vi "Periodic Tasks.vi"(8 "error in":errorcluster) -> ()   [LabVIEW 2014]
doc: "This VI runs in parallel to other tasks. It can contain as many user-defined periodic loops as you need. These can carry out PID or other sorts of timed response."
uses:
  <vilib>/Rock Robotics/WPI/Relay/WPI_RelayValue.ctl
  <vilib>/Rock Robotics/SystemInterfaces/Utilities/FPGA_UtilitiesLED Source.ctl
  <vilib>/Rock Robotics/SystemInterfaces/Utilities/FPGA_UtilitiesLED State.ctl
  <vilib>/Rock Robotics/WPI/DriverStation/WPI_DriverStationRobotMode2.ctl
  <vilib>/Rock Robotics/WPI/Compressor/WPI_CompressorGetSetRefNum.vi
  Robot Global Data.vi
  <vilib>/Rock Robotics/WPI/Solenoid/Deprecated/WPI_SolenoidSetBool.vi
panel:
  out "Passing Ball":bool
  out "kicker was on":bool
  out "Lights Relay Indicator":T1
  out "pickup arm motor shooting":bool
  out "Gate shooting":bool
  out "Catapult Switch Triggered":bool
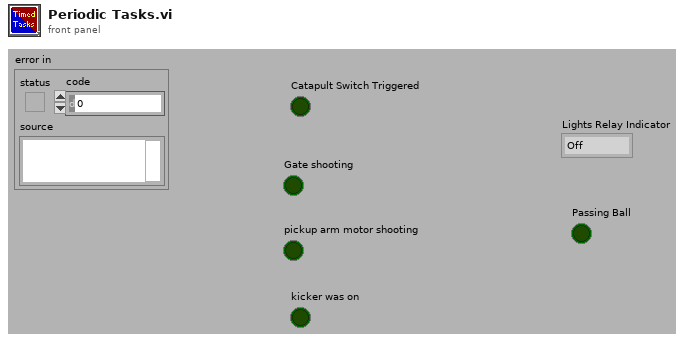
[diagram p1: front panel]
types:
  T1 = typedef "WPI_RelayValue.ctl" = enum16{"Off", "On", "Forward", "Reverse"}
  T2 = typedef "WPI_RelayDevRef.ctl" = cluster{"DevStatus":errorcluster, "Relay Channel":T3, "Digital Module":T4, "Relay Direction":T5}
  T3 = typedef "FPGA_DIORelayChannel.ctl" = enum8{"Relay 1", "Relay 2", "Relay 3", "Relay 4", "Relay 5", "Relay 6", "Relay 7", "Relay 8", "Invalid"}
  T4 = typedef "FPGA_TypedefDigitalModule.ctl" = enum16{"Digital Module 1", "Digital Module 2"}
  T5 = typedef "WPI_RelayDirection.ctl" = enum16{"Both directions", "Forward only", "Reverse only"}
  T6 = typedef "WPI_DigitalInputDevRef.ctl" = cluster{"DevStatus":errorcluster, "DIO Channel":T7, "Digital Module":T4}
  T7 = typedef "FPGA_DIOChannel.ctl" = enum8{"DIO 1", "DIO 2", "DIO 3", "DIO 4", "DIO 5", "DIO 6", "DIO 7", "DIO 8", "DIO 9", "DIO 10", "DIO 11", "DIO 12", "DIO 13", "DIO 14", "Invalid"}
  T8 = typedef "WPI_SolenoidDevRef.ctl" = cluster{"DevStatus":errorcluster, "Solenoid Module":T9, "Forward Solenoid Channel":T10, "Reverse Solenoid Channel":T10}
  T9 = typedef "FPGA_TypedefSolenoidModule.ctl" = enum16{"Solenoid Module 1", "Solenoid Module 2"}
  T10 = typedef "WPI_SolenoidChannel.ctl" = enum8{"Solenoid 1", "Solenoid 2", "Solenoid 3", "Solenoid 4", "Solenoid 5", "Solenoid 6", "Solenoid 7", "Solenoid 8", "Invalid"}
  T11 = typedef "WPI_MotorControlDeviceRef.ctl" = cluster{"DeviceStatus":errorcluster, "Type":enum16{"PWM", "CAN"}, "PWM":cluster{"Digital Module":T4, "PWM Channel":T12, "DeadBand":T13}, "CAN":cluster{"Device Number":u8, "Control Mode":T14, "Semaphore":T15, "Max Vout":dbl}, "Invert":bool, "TransformRef":T16, "InvTransformRef":T16}
  T12 = typedef "FPGA_DIOPWMChannel.ctl" = enum8{"PWM 1", "PWM 2", "PWM 3", "PWM 4", "PWM 5", "PWM 6", "PWM 7", "PWM 8", "PWM 9", "PWM 10", "Invalid"}
  T13 = typedef "WPI_PWMDeadband.ctl" = cluster{"Name":string, "maxPositivePwm":i32, "minPositivePwm":i32, "centerPwm":i32, "maxNegativePwm":i32, "minNegativePwm":i32, "angularRange":u16}
  T14 = typedef "WPI_CANJaguar_ControlMode.ctl" = enum8{"Percent VBus", "Current", "Speed", "Position", "Voltage"}
  T15 = typedef "Semaphore RefNum" = refnum<k1>
  T16 = typedef "WPI_PWMTransform_ConPane.ctl" = refnum<vi>
  T17 = typedef "WPI_AnalogChannelDevRef.ctl" = cluster{"DevStatus":errorcluster, "Analog Module":T18, "Analog Channel":T19}
  T18 = typedef "FPGA_TypedefAnalogModule.ctl" = enum16{"Analog Module 1", "Analog Module 2"}
  T19 = typedef "FPGA_AIChannel.ctl" = enum8{"AI 1", "AI 2", "AI 3", "AI 4", "AI 5", "AI 6", "AI 7", "AI 8", "Invalid"}
  T20 = typedef "FPGA_UtilitiesLED State.ctl" = enum16{"Off", "On", "Toggle"}
  T21 = typedef "FPGA_UtilitiesLED Source.ctl" = enum16{"User LED", "FPGA LED"}
  T22 = typedef "WPI_DriverStationRobotMode2.ctl" = enum16{"Autonomous Disabled", "Autonomous Enabled", "Teleop Disabled", "Teleop Enabled", "Disconnected", "Finish", "Test Disabled", "Test Enabled"}
  T23 = typedef "WPI_CompressorDevRef.ctl" = cluster{"DevStatus":errorcluster, "DigitalInputDevRef":T6, "RelayDevRef":T2}
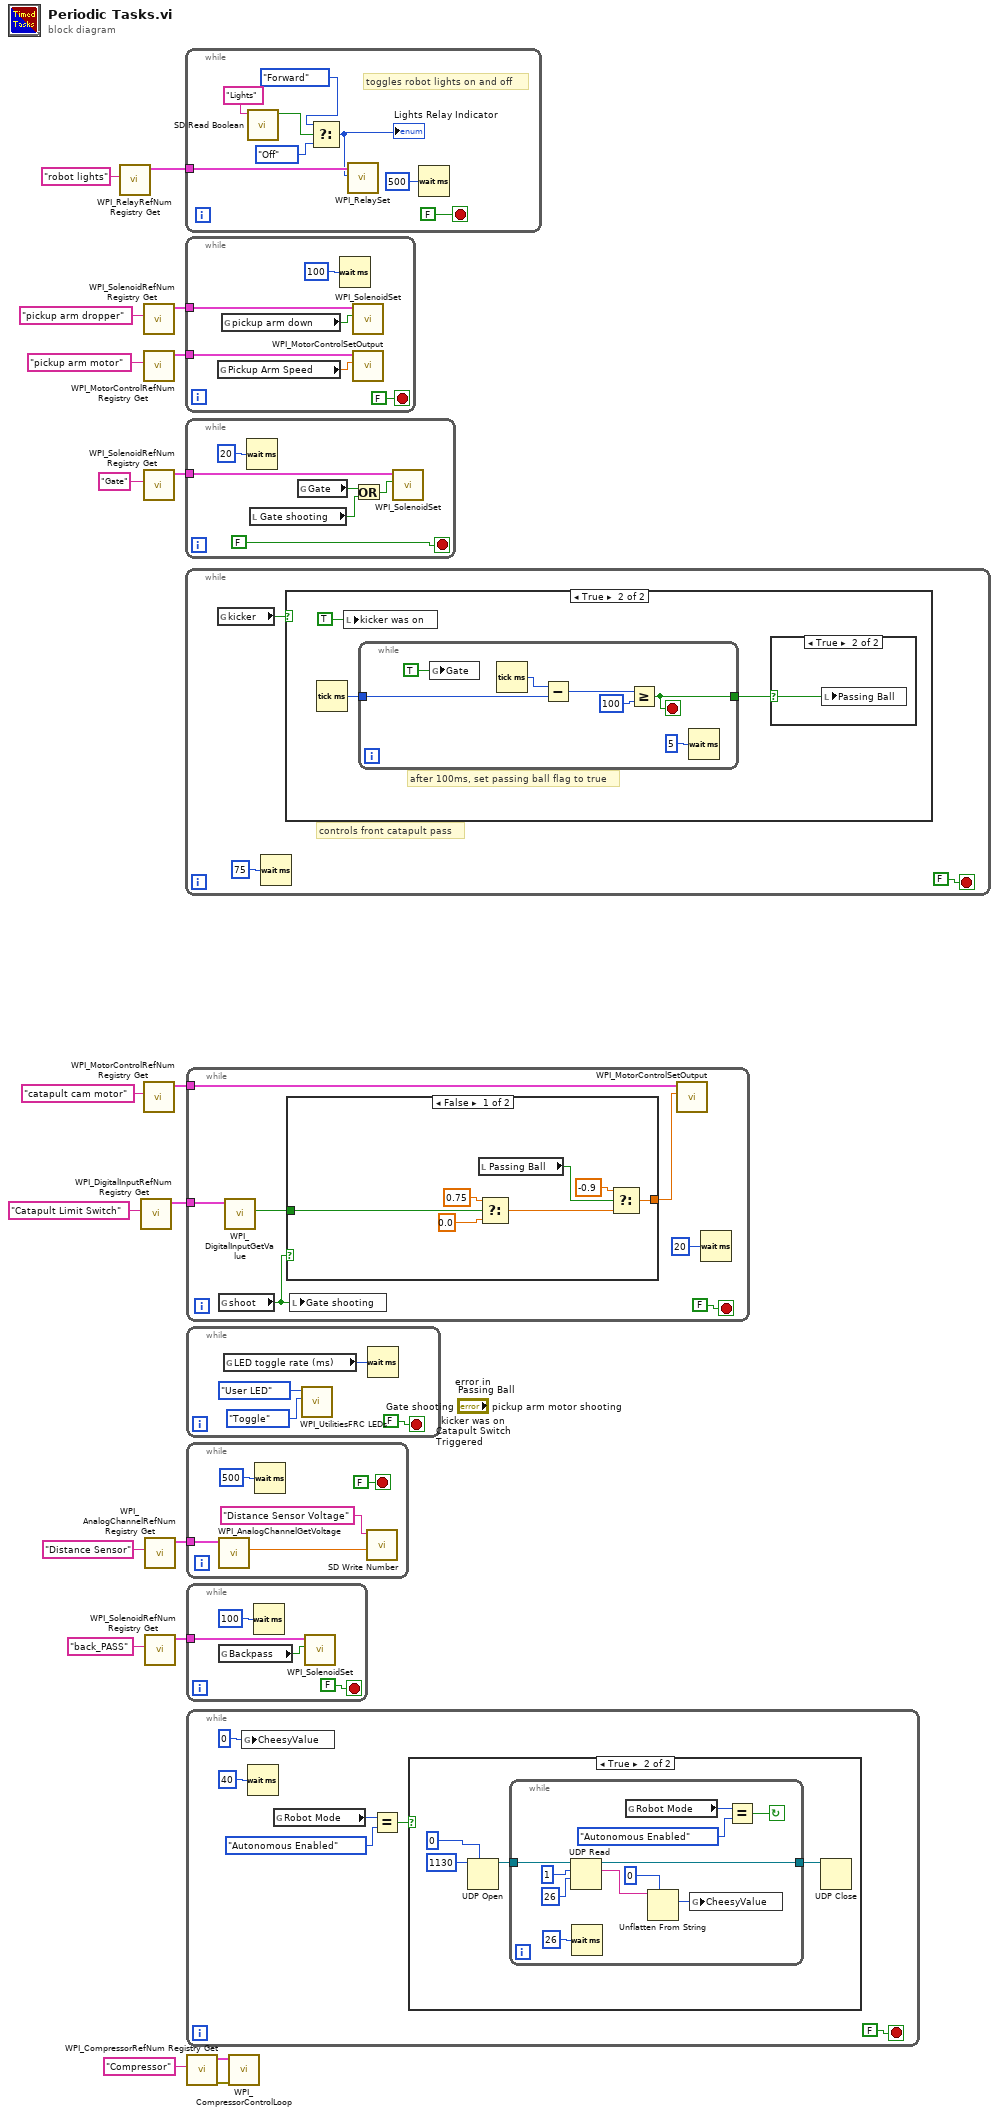
[diagram p0: block diagram]
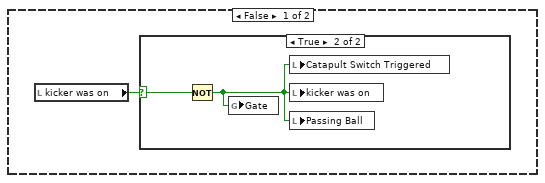
[diagram p3: hidden frame]
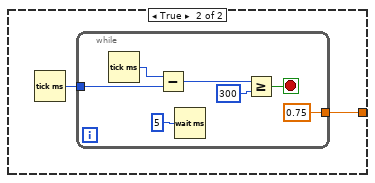
[diagram p6: hidden frame]
diagram:
  n1 = call <vilib>:"WPI_RelayRefNum Registry Get.vi"("refnum name"="robot lights") -> ("RelayDevRef"=w6:T2)  [unwired: 9 in, 1 out]
  n2 = call <vilib>:"WPI_DigitalInputRefNum Registry Get.vi"("refnum name"="Catapult Limit Switch") -> ("DigitalInputDevRef"=w8:T6)  [unwired: 9 in, 1 out]
  n3 = call <vilib>:"WPI_SolenoidRefNum Registry Get.vi"("refnum name"="pickup arm dropper") -> ("SolenoidDevRef"=w12:T8)  [unwired: 9 in, 1 out]
  n4 = call <vilib>:"WPI_MotorControlRefNum Registry Get.vi"("refnum name"="pickup arm motor") -> ("MotorControlDevRef"=w10:T11)  [unwired: 9 in, 1 out]
  n5 = call <vilib>:"WPI_SolenoidRefNum Registry Get.vi"("refnum name"="Gate") -> ("SolenoidDevRef"=w5:T8)  [unwired: 9 in, 1 out]
  n6 = call <vilib>:"WPI_MotorControlRefNum Registry Get.vi"("refnum name"="catapult cam motor") -> ("MotorControlDevRef"=w15:T11)  [unwired: 9 in, 1 out]
  n7 = call <vilib>:"WPI_AnalogChannelRefNum Registry Get.vi"("refnum name"="Distance Sensor") -> ("AIDeviceRef"=w1:T17)  [unwired: 9 in, 1 out]
  n8 = call <vilib>:"WPI_SolenoidRefNum Registry Get.vi"("refnum name"="back_PASS") -> ("SolenoidDevRef"=w3:T8)  [unwired: 9 in, 1 out]
  n9 = while {
    tunnel: w6 -> [w24]
    stop <- FALSE stop-if-true
    # "toggles robot lights on and off"
    n10 = call <vilib>:"SD Read Boolean.vi"("Name"="Lights") -> ("Boolean"=w23:bool)  [unwired: 8 in, 2 out]
    n11 = Select(t=WPI_RelayValue."Forward" ("RelayValue"), s=w23, f=WPI_RelayValue."Off" ("RelayValue")) -> (s? t:f=w20:T1)
    "Lights Relay Indicator" <- w20
    n12 = call <vilib>:"WPI_RelaySet.vi"("RelayValue"=w20, "RelayDevRef"=w24) -> ()  [unwired: 8 in, 2 out]
    n13 = Wait (ms)(milliseconds to wait=u32 500) -> ()  [unwired: 1 out]
  }
  n14 = while {
    tunnel: w12 -> [w33]
    tunnel: w10 -> [w32]
    stop <- FALSE stop-if-true
    n15 = global read "Robot Global Data.vi" "Pickup Arm Speed"() -> (w29:dbl)
    n16 = global read "Robot Global Data.vi" "pickup arm down"() -> (w28:bool)
    n17 = Wait (ms)(milliseconds to wait=u32 100) -> ()  [unwired: 1 out]
    n18 = call-poly <vilib>:"WPI_SolenoidSet.vi"("Value"=w28, "SolenoidDevRef"=w33) -> ()  [unwired: 8 in, 2 out]
    n19 = call <vilib>:"WPI_MotorControlSetOutput.vi"("Output"=w29, "MotorControlDevRef"=w32) -> ()  [unwired: 7 in, 3 out]
  }
  n20 = while {
    tunnel: w5 -> [w35]
    stop <- FALSE stop-if-true
    n21 = Wait (ms)(milliseconds to wait=u32 20) -> ()  [unwired: 1 out]
    n22 = local read "Gate shooting"() -> (w39:bool)
    n23 = global read "Robot Global Data.vi" "Gate"() -> (w38:bool)
    n24 = Or(x=w38, y=w39) -> (x .or. y?=w34:bool)
    n25 = call-poly <vilib>:"WPI_SolenoidSet.vi"("Value"=w34, "SolenoidDevRef"=w35) -> ()  [unwired: 8 in, 2 out]
  }
  n26 = while {
    stop <- FALSE stop-if-true
    # "controls front catapult pass"
    n27 = global read "Robot Global Data.vi" "kicker"() -> (w40:bool)
    n28 = Wait (ms)(milliseconds to wait=u32 75) -> ()  [unwired: 1 out]
    n29 = case shown="True" w40 {
      frame False {
        n30 = local read "kicker was on"() -> (w43:bool)
        n31 = case shown="True" w43 {
          selector: w43 -> [_ w45]
          frame False {
          }
          frame True {
            n32 = Not(x=w45) -> (.not. x?=w44:bool)
            n33 = global write "Robot Global Data.vi" "Gate"(w44) -> ()
            n34 = local write "Catapult Switch Triggered"(w44) -> ()
            n35 = local write "kicker was on"(w44) -> ()
            n36 = local write "Passing Ball"(w44) -> ()
          }
        }
      }
      frame True {
        # "after 100ms, set passing ball flag to true"
        n37 = Tick Count (ms)() -> (millisecond timer value=w47:u32)
        n38 = local write "kicker was on"(TRUE ("kicker was on")) -> ()
        n39 = while {
          tunnel: w47 -> [w55]
          tunnel: [w50] -> w46
          stop <- w50 stop-if-true
          n40 = global write "Robot Global Data.vi" "Gate"(TRUE ("Gate")) -> ()
          n41 = Tick Count (ms)() -> (millisecond timer value=w54:u32)
          n42 = Subtract(x=w54, y=w55) -> (x-y=w53:u32)
          n43 = Greater Or Equal?(x=w53, y=u32 100) -> (x >= y?=w50:bool)
          n44 = Wait (ms)(milliseconds to wait=u32 5) -> ()  [unwired: 1 out]
        }
        n45 = case shown="True" w46 {
          selector: w46 -> [_ w56]
          frame False {
          }
          frame True {
            n46 = local write "Passing Ball"(w56) -> ()
          }
        }
      }
    }
  }
  n47 = while {
    tunnel: w15 -> [w61]
    tunnel: w8 -> [w59]
    stop <- FALSE stop-if-true
    n48 = global read "Robot Global Data.vi" "shoot"() -> (w57:bool)
    n49 = call <vilib>:"WPI_DigitalInputGetValue.vi"("DigitalInputDevRef"=w59) -> ("Value"=w58:bool)  [unwired: 8 in, 2 out]
    n50 = case shown="False" w57 {
      tunnel: [w70 w71] -> w60
      tunnel: w58 -> [w64 _]
      frame False {
        n51 = local read "Passing Ball"() -> (w69:bool)
        n52 = Select(t=0.75 ("f"), s=w64, f=0.0 ("t")) -> (s? t:f=w67:dbl)
        n53 = Select(t=-0.9, s=w69, f=w67) -> (s? t:f=w70:dbl)
      }
      frame True {
        n54 = Tick Count (ms)() -> (millisecond timer value=w72:u32)
        n55 = while {
          tunnel: [0.75 ("Output")] -> w71
          tunnel: w72 -> [w77]
          stop <- w74 stop-if-true
          n56 = Tick Count (ms)() -> (millisecond timer value=w78:u32)
          n57 = Subtract(x=w78, y=w77) -> (x-y=w73:u32)
          n58 = Wait (ms)(milliseconds to wait=u32 5) -> ()  [unwired: 1 out]
          n59 = Greater Or Equal?(x=w73, y=u32 300) -> (x >= y?=w74:bool)
        }
      }
    }
    n60 = local write "Gate shooting"(w57) -> ()
    n61 = call <vilib>:"WPI_MotorControlSetOutput.vi"("Output"=w60, "MotorControlDevRef"=w61) -> ()  [unwired: 7 in, 3 out]
    n62 = Wait (ms)(milliseconds to wait=u32 20) -> ()  [unwired: 1 out]
  }
  n63 = while {
    stop <- FALSE stop-if-true
    n64 = global read "Robot Global Data.vi" "LED toggle rate (ms)"() -> (w80:u32)
    n65 = call <vilib>:"WPI_UtilitiesFRC LEDs.vi"("State"=FPGA_UtilitiesLED_State."Toggle", "LED Type"=FPGA_UtilitiesLED_Source."User LED") -> ()  [unwired: 1 in, 9 out]
    n66 = Wait (ms)(milliseconds to wait=w80) -> ()  [unwired: 1 out]
  }
  n67 = while {
    tunnel: w1 -> [w86]
    stop <- FALSE stop-if-true
    n68 = call <vilib>:"WPI_AnalogChannelGetVoltage.vi"("AIDeviceRef"=w86) -> ("Voltage"=w85:dbl)  [unwired: 8 in, 2 out]
    n69 = Wait (ms)(milliseconds to wait=u32 500) -> ()  [unwired: 1 out]
    n70 = call <vilib>:"SD Write Number.vi"("Numeric"=w85, "Name"="Distance Sensor Voltage") -> ()  [unwired: 8 in, 2 out]
  }
  n71 = while {
    tunnel: w3 -> [w90]
    stop <- FALSE stop-if-true
    n72 = global read "Robot Global Data.vi" "Backpass"() -> (w89:bool)
    n73 = Wait (ms)(milliseconds to wait=u32 100) -> ()  [unwired: 1 out]
    n74 = call-poly <vilib>:"WPI_SolenoidSet.vi"("Value"=w89, "SolenoidDevRef"=w90) -> ()  [unwired: 8 in, 2 out]
  }
  n75 = while {
    stop <- FALSE stop-if-true
    n76 = global write "Robot Global Data.vi" "CheesyValue"(u8 0 ("CheesyValue")) -> ()
    n77 = Wait (ms)(milliseconds to wait=u32 40) -> ()  [unwired: 1 out]
    n78 = global read "Robot Global Data.vi" "Robot Mode"() -> (w94:T22)
    n79 = Equal?(x=w94, y=WPI_DriverStationRobotMode2."Autonomous Enabled" ("Robot Mode")) -> (x = y?=w96:bool)
    n80 = case shown="True" w96 {
      frame False {
      }
      frame True {
        n81 = UDP Open(7:u32 0 ("net address"), 11:u16 1130 ("port")) -> (port=w101:refnum<k16>)  [unwired: 3 in, 2 out]
        n82 = while {
          tunnel: w101 -> [w113]
          tunnel: [w105] -> w102
          stop <- w106 continue-if-true
          n83 = UDP Read(connection ID=w113, max size (548)=1, timeout ms (25000)=26) -> (data out=w112:string, 3:w105:refnum<k16>)  [unwired: 1 in, 3 out]
          n84 = Wait (ms)(milliseconds to wait=u32 26) -> ()  [unwired: 1 out]
          n85 = global read "Robot Global Data.vi" "Robot Mode"() -> (w104:T22)
          n86 = Unflatten From String(type=u8 0, binary string=w112) -> (value=w103:u8)  [unwired: 3 in, 2 out]
          n87 = global write "Robot Global Data.vi" "CheesyValue"(w103) -> ()
          n88 = Equal?(x=w104, y=WPI_DriverStationRobotMode2."Autonomous Enabled" ("Robot Mode")) -> (x = y?=w106:bool)
        }
        n89 = UDP Close(connection ID=w102) -> ()  [unwired: 1 in, 2 out]
      }
    }
  }
  n90 = call <vilib>:"WPI_CompressorRefNum Registry Get.vi"("refnum name"="Compressor") -> ("error out"=w18:errorcluster, "CompressorDevRef"=w17:T23)  [unwired: 9 in]
  n91 = call <vilib>:"WPI_CompressorControlLoop.vi"("error in (no error)"=w18, "CompressorDevRef"=w17) -> ()  [unwired: 10 in]
